vi "Create_equidistant_array.vi"(10 "Elapsed Time (s)":dbl[](array[numeric]), 11 "dt (s)":dbl) -> (3 "Array":dbl[](array[numeric]))   [LabVIEW 2015]
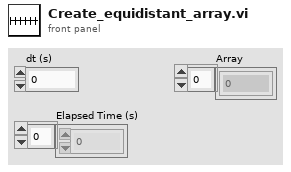
[diagram p1: front panel]
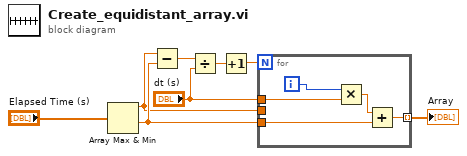
[diagram p0: block diagram]
diagram:
  n1 = Array Max & Min(array="Elapsed Time (s)") -> (max value=w4:dbl, min value=w5:dbl)  [unwired: 2 out]
  n2 = Subtract(x=w4, y=w5) -> (x-y=w6:dbl)
  n3 = Divide(x=w6, y="dt (s)") -> (x/y=w2:dbl)
  n4 = Increment(x=w2) -> (x+1=w3:dbl)
  n5 = for {
    N: w3 -> [_]
    tunnel: w5 -> [w10]
    tunnel: w4 -> [_]
    tunnel: [w12] -> w8 mode=indexing
    tunnel: "dt (s)" -> [w11]
    i -> [w9]
    n6 = Multiply(x=w9, y=w11) -> (x*y=w13:dbl)
    n7 = Add(x=w13, y=w10) -> (x+y=w12:dbl)
  }
  "Array" <- w8
